vi "test.vi"() -> ()   [LabVIEW 2010]
uses:
  common/classes/Image/Image/Image.lvclass
  common/classes/Image/Image/target_format_enum.ctl
panel:
  out "Elapsed Time (sec)":dbl format="%0.3f"
  in  "quit":bool
  in  "stop":bool
  out "Image":T1(plugin-control)
  out "error out":errorcluster
  in  "error in (no error)":errorcluster
  in  "save":bool
  in  "load":bool
  in  "Image.lvclass":refnum<class "Image.lvclass">
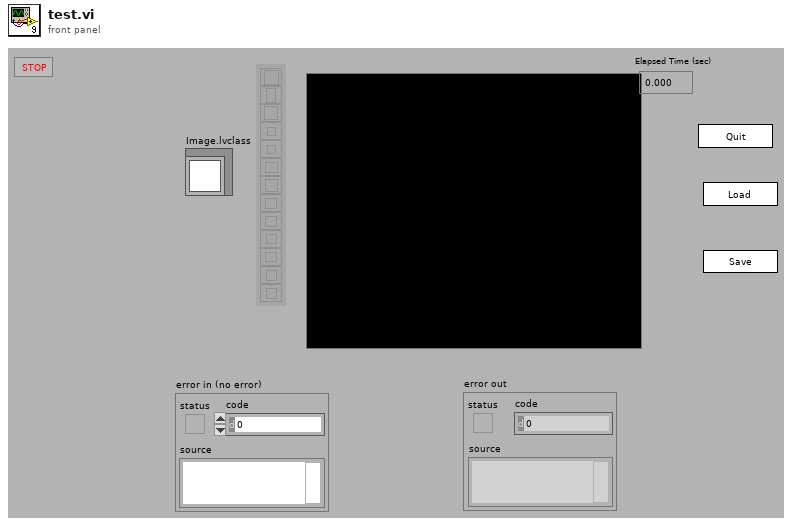
[diagram p1: front panel]
types:
  T1 = typedef "IMAQ Image.ctl" = refnum<image>
  T2 = typedef "target_format_enum.ctl" = enum16{"don't force", "uint8", "uint16", "int16", "uint32", "int32", "single float"}
  T3 = typedef "Image Type" = u32
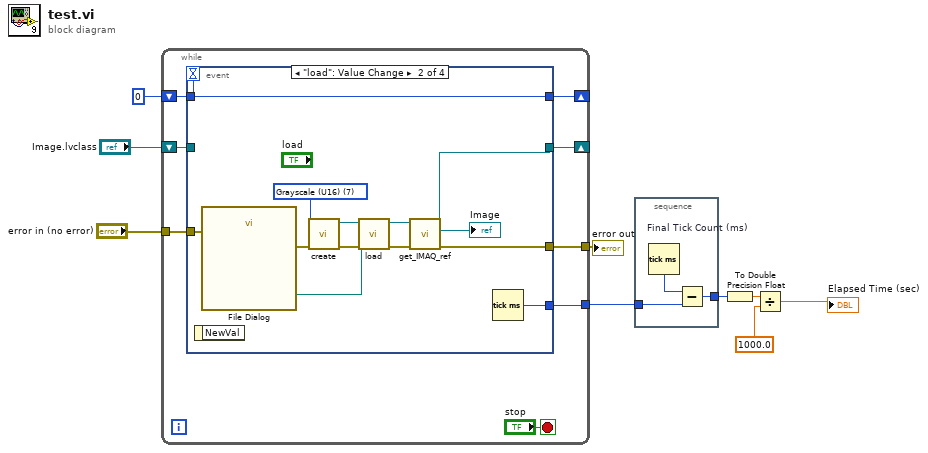
[diagram p0: block diagram]
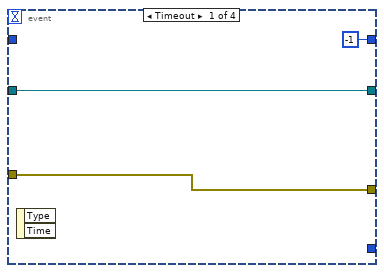
[diagram p2: hidden frame]
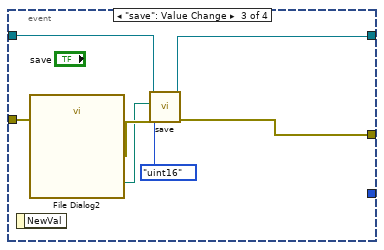
[diagram p3: hidden frame]
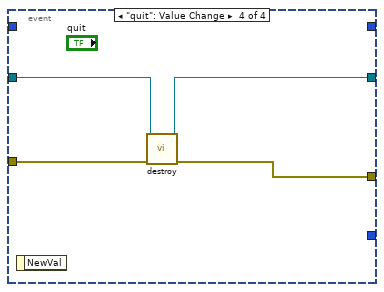
[diagram p4: hidden frame]
diagram:
  n1 = while {
    tunnel: "error in (no error)" -> [w17]
    tunnel: [w16] -> w8
    shift-right: [w13] -> _
    shift-left: "Image.lvclass" -> [w14]
    shift-right: [w12] -> _
    shift-left: 0 -> [w11]
    tunnel: [w10] -> w4
    stop <- "stop" stop-if-true
    n2 = event shown="[1] \"load\": Value Change" {
      selector: _ -> [_ _ _ _]
      dyn-events: _ -> [_ _ _ _]
      timeout: w11 -> [_ _ _ _]
      tunnel: w17 -> [w19 w31 w36 w44]
      tunnel: [w19 w25 w38 w43] -> w16
      tunnel: w14 -> [w20 _ w40 w42]
      tunnel: [w20 w23 w37 w41] -> w13
      tunnel: w11 -> [_ w22 _ _]
      tunnel: [-1 w22 _ _] -> w12
      tunnel: [_ w21 _ _] -> w10
      event Timeout {
        n3 = event-data() -> ()  [unwired: 1 in, 2 out]
      }
      event "load": Value Change {
        w33 = T3 7 items=["Grayscale (U8)", "Grayscale (I16)", "Grayscale (SGL)", "Complex (CSG)", "RGB (U32)", "HSL (U32)", "RGB (U64)", "Grayscale (U16)"] ("Image Type")
        n4 = event-data() -> ()  [unwired: 1 in, 1 out]
        n5 = call "File Dialog"("error in"=w31) -> ("selected path"=w30:path, "error out"=w28:errorcluster)  [unwired: 11 in, 2 out]
        n6 = call "create.vi"("error in (no error)"=w28, "Image Type"=w33) -> ("error out"=w29:errorcluster, "Image out"=w32:refnum<class "Image.lvclass">)  [unwired: 8 in]
        n7 = call-dynamic "load.vi"("error in (no error)"=w29, "Path"=w30, "Image in"=w32) -> ("error out"=w27:errorcluster, "Image out"=w24:refnum<class "Image.lvclass">)  [unwired: 5 in, 2 out]
        n8 = call-dynamic "get_IMAQ_ref.vi"("error in (no error)"=w27, "Image.lvclass in"=w24) -> ("error out"=w25:errorcluster, "Image"=→"Image":T1, "Image.lvclass out"=w23:refnum<class "Image.lvclass">)  [unwired: 5 in, 2 out]
        n9 = Tick Count (ms)() -> (millisecond timer value=w21:u32)
      }
      event "save": Value Change {
        n10 = event-data() -> ()  [unwired: 1 in, 1 out]
        n11 = call "File Dialog2"("error in"=w36) -> ("selected path"=w34:path, "error out"=w35:errorcluster)  [unwired: 11 in, 2 out]
        n12 = call "save.vi"("error in (no error)"=w35, "force format?"=target_format_enum."uint16", "path"=w34, "Image in"=w40) -> ("error out"=w38:errorcluster, "Image out"=w37:refnum<class "Image.lvclass">)  [unwired: 6 in]
      }
      event "quit": Value Change {
        n13 = event-data() -> ()  [unwired: 1 in, 1 out]
        n14 = call-dynamic "destroy.vi"("error in (no error)"=w44, "Image in"=w42) -> ("error out"=w43:errorcluster, "Image out"=w41:refnum<class "Image.lvclass">)  [unwired: 8 in]
      }
    }
  }
  "error out" <- w8
  n15 = stacked-sequence {
    tunnel: w4 -> [w47]
    tunnel: [w45] -> w1
    frame #0 {
      n16 = Tick Count (ms) "Final Tick Count (ms)"() -> (millisecond timer value=w46:u32)
      n17 = Subtract(x=w46, y=w47) -> (x-y=w45:u32)
    }
  }
  n18 = To Double Precision Float(number=w1) -> (double precision float=w2:dbl)
  n19 = Divide(x=w2, y=1000.0) -> (x/y=→"Elapsed Time (sec)":dbl)
